vi "Count_if_Subtrack_Is_Enough_for_Cost_F()-3.vi"(3 "[IN] Indexes for Jumps\nfrom Previous Origin":i32[](array[numeric]), 4 "[IN] Index of Problem \nPoint Inside Track":i32, 5 "[IN] Minimal Subtrack Length \n(Points without problems) for\nMaking Desicion":i32, 6 "[IN] Dot Statuses in Track":i16[](array[numeric])) -> (1 "[OUT] Index of Last \nPoint in Track":i32, 2 "[OUT] It's enough to make\nconclusion using subtrack":bool)   [LabVIEW 2013]
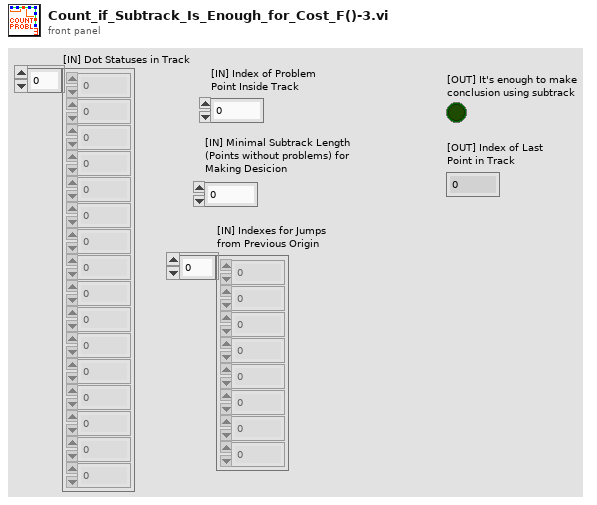
[diagram p1: front panel]
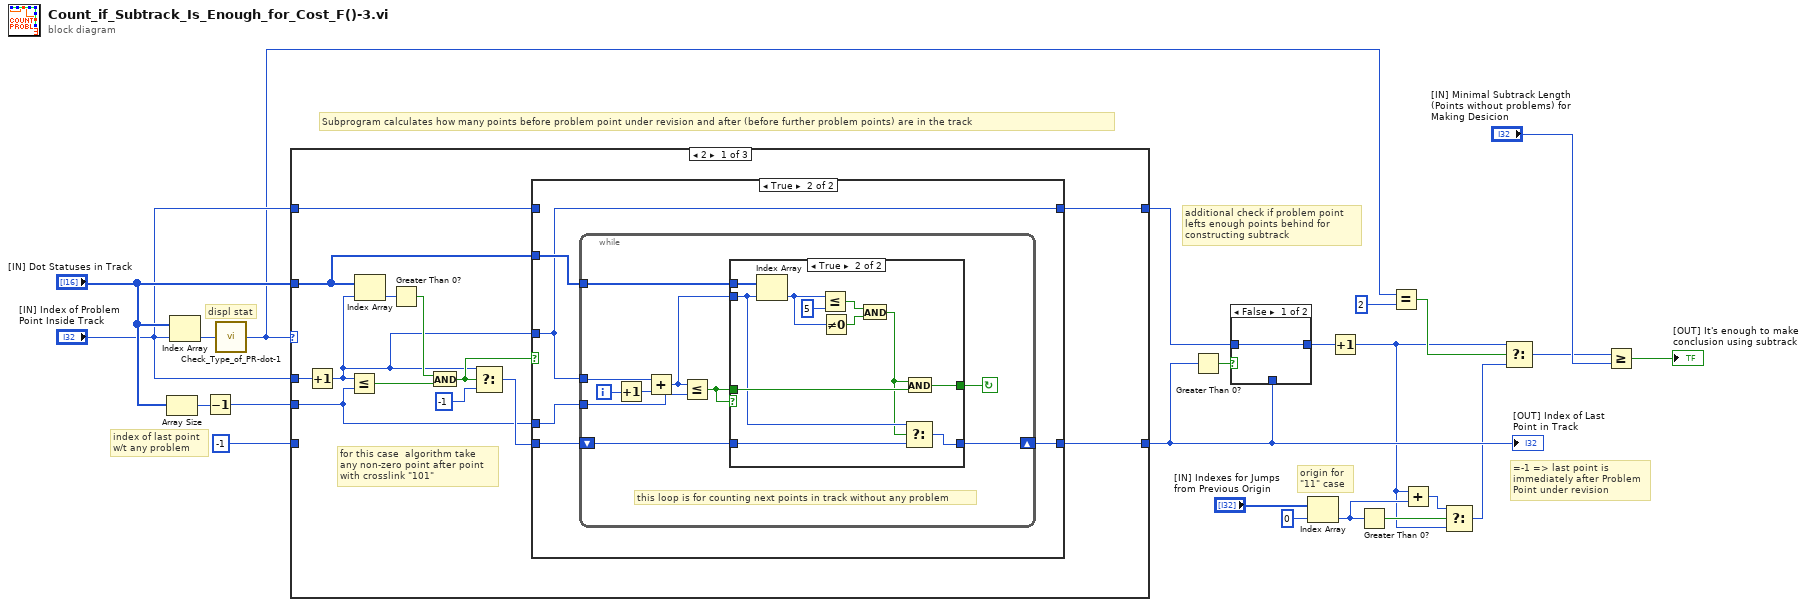
[diagram p0: block diagram]
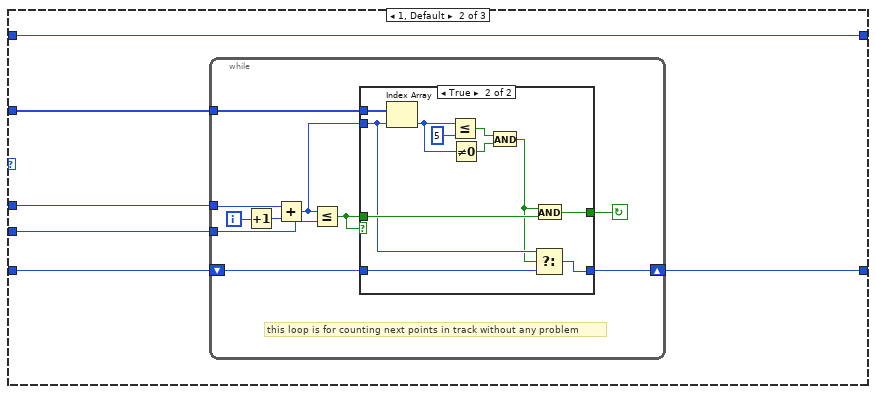
[diagram p4: hidden frame]
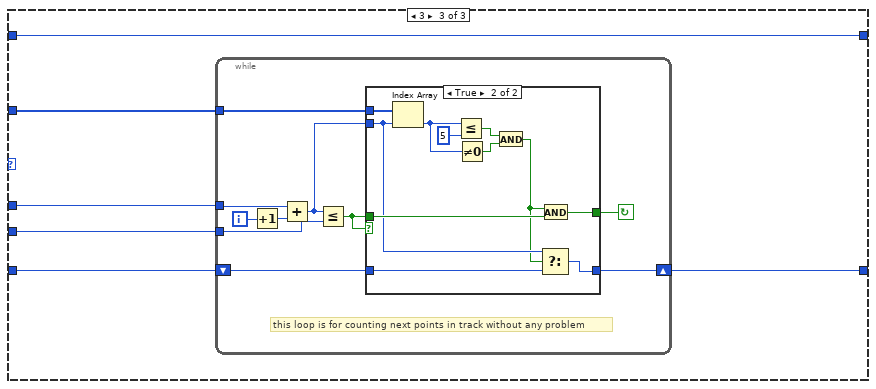
[diagram p6: hidden frame]
diagram:
  # "origin for \n\"11\" case"
  # "displ stat"
  # "additional check if problem point \nlefts enough points behind for \nconstructing subtrack"
  # "=-1 => last point is\nimmediately after Problem \nPoint under revision"
  # "Subprogram calculates how many points before problem point under revision and after (before further problem points) are in the track"
  # "index of last point\nw/t any problem"
  n1 = Array Size(array="[IN] Dot Statuses in Track") -> (size(s)=w23:i32)
  n2 = Index Array(array="[IN] Dot Statuses in Track", index="[IN] Index of Problem \nPoint Inside Track") -> (element=w15:i16)
  n3 = Decrement(x=w23) -> (x-1=w22:i32)
  n4 = call "Check_Type_of_PR-dot-1.vi"("[IN] dot status"=w15) -> ("[OUT] Type of\nproblem dot"=w10:i32)
  n5 = case shown="2" w10 {
    tunnel: w22 -> [w26 w72 w99]
    tunnel: -1 -> [_ w71 w98]
    tunnel: [w27 w70 w97] -> w17
    tunnel: "[IN] Dot Statuses in Track" -> [w28 w69 w101]
    tunnel: "[IN] Index of Problem \nPoint Inside Track" -> [w36 w68 w100]
    tunnel: "[IN] Index of Problem \nPoint Inside Track" -> [w24 w67 w96]
    tunnel: [w25 w67 w96] -> w13
    frame 2 {
      # "for this case  algorithm take\nany non-zero point after point\nwith crosslink \"101\""
      n6 = Increment(x=w36) -> (x+1=w29:i32)
      n7 = Less Or Equal?(x=w29, y=w26) -> (x <= y?=w34:bool)
      n8 = Index Array(array=w28, index=w29) -> (element=w35:i16)
      n9 = Greater Than 0?(x=w35) -> (x > 0?=w33:bool)
      n10 = And(x=w33, y=w34) -> (x .and. y?=w31:bool)
      n11 = Select(t=w29, s=w31, f=-1) -> (s? t:f=w30:i32)
      n12 = case shown="True" w31 {
        tunnel: w30 -> [w38 w43]
        tunnel: w29 -> [_ w39]
        tunnel: w28 -> [_ w42]
        tunnel: [w38 w41] -> w27
        tunnel: w26 -> [_ w40]
        tunnel: [w37 w39] -> w25
        tunnel: w24 -> [w37 _]
        frame False {
        }
        frame True {
          n13 = while {
            tunnel: w40 -> [w51]
            tunnel: w39 -> [w44]
            tunnel: w42 -> [w50]
            shift-right: [w45] -> w41
            shift-left: w43 -> [w46]
            i -> [w53]
            stop <- w47 continue-if-true
            # "this loop is for counting next points in track without any problem"
            n14 = Increment(x=w53) -> (x+1=w52:i32)
            n15 = Add(x=w44, y=w52) -> (x+y=w49:i32)
            n16 = Less Or Equal?(x=w49, y=w51) -> (x <= y?=w48:bool)
            n17 = case shown="True" w48 {
              tunnel: w50 -> [_ w66]
              tunnel: w49 -> [_ w57]
              tunnel: w48 -> [w55 w60]
              tunnel: [w55 w61] -> w47
              tunnel: w46 -> [w54 w58]
              tunnel: [w54 w59] -> w45
              frame False {
                # "it's last point in subtrack"
              }
              frame True {
                n18 = Index Array(array=w66, index=w57) -> (element=w64:i16)
                n19 = Less Or Equal?(x=w64, y=i16 5) -> (x <= y?=w63:bool)
                n20 = Not Equal To 0?(x=w64) -> (x != 0?=w62:bool)
                n21 = And(x=w63, y=w62) -> (x .and. y?=w56:bool)
                n22 = Select(t=w57, s=w56, f=w58) -> (s? t:f=w59:i32)
                n23 = And(x=w56, y=w60) -> (x .and. y?=w61:bool)
              }
            }
          }
        }
      }
    }
    frame 1, Default {
      n24 = while {
        tunnel: w72 -> [w80]
        tunnel: w68 -> [w73]
        tunnel: w69 -> [w79]
        shift-right: [w74] -> w70
        shift-left: w71 -> [w75]
        i -> [w82]
        stop <- w76 continue-if-true
        # "this loop is for counting next points in track without any problem"
        n25 = Increment(x=w82) -> (x+1=w81:i32)
        n26 = Add(x=w73, y=w81) -> (x+y=w78:i32)
        n27 = Less Or Equal?(x=w78, y=w80) -> (x <= y?=w77:bool)
        n28 = case shown="True" w77 {
          tunnel: w79 -> [_ w95]
          tunnel: w78 -> [_ w86]
          tunnel: w77 -> [w84 w89]
          tunnel: [w84 w90] -> w76
          tunnel: w75 -> [w83 w87]
          tunnel: [w83 w88] -> w74
          frame False {
            # "it's last point in subtrack"
          }
          frame True {
            n29 = Index Array(array=w95, index=w86) -> (element=w93:i16)
            n30 = Less Or Equal?(x=w93, y=i16 5) -> (x <= y?=w92:bool)
            n31 = Not Equal To 0?(x=w93) -> (x != 0?=w91:bool)
            n32 = And(x=w92, y=w91) -> (x .and. y?=w85:bool)
            n33 = Select(t=w86, s=w85, f=w87) -> (s? t:f=w88:i32)
            n34 = And(x=w85, y=w89) -> (x .and. y?=w90:bool)
          }
        }
      }
    }
    frame 3 {
      n35 = while {
        tunnel: w99 -> [w109]
        tunnel: w100 -> [w102]
        tunnel: w101 -> [w108]
        shift-right: [w103] -> w97
        shift-left: w98 -> [w104]
        i -> [w111]
        stop <- w105 continue-if-true
        # "this loop is for counting next points in track without any problem"
        n36 = Increment(x=w111) -> (x+1=w110:i32)
        n37 = Add(x=w102, y=w110) -> (x+y=w107:i32)
        n38 = Less Or Equal?(x=w107, y=w109) -> (x <= y?=w106:bool)
        n39 = case shown="True" w106 {
          tunnel: w108 -> [_ w124]
          tunnel: w107 -> [_ w115]
          tunnel: w106 -> [w113 w118]
          tunnel: [w113 w119] -> w105
          tunnel: w104 -> [w112 w116]
          tunnel: [w112 w117] -> w103
          frame False {
            # "it's last point in subtrack"
          }
          frame True {
            n40 = Index Array(array=w124, index=w115) -> (element=w122:i16)
            n41 = Less Or Equal?(x=w122, y=i16 5) -> (x <= y?=w121:bool)
            n42 = Not Equal To 0?(x=w122) -> (x != 0?=w120:bool)
            n43 = And(x=w121, y=w120) -> (x .and. y?=w114:bool)
            n44 = Select(t=w115, s=w114, f=w116) -> (s? t:f=w117:i32)
            n45 = And(x=w114, y=w118) -> (x .and. y?=w119:bool)
          }
        }
      }
    }
  }
  "[OUT] Index of Last \nPoint in Track" <- w17
  n46 = Greater Than 0?(x=w17) -> (x > 0?=w19:bool)
  n47 = case shown="False" w19 {
    tunnel: w13 -> [w125 _]
    tunnel: [w125 w126] -> w18
    tunnel: w17 -> [_ w126]
    frame False {
    }
    frame True {
    }
  }
  n48 = Index Array(array="[IN] Indexes for Jumps\nfrom Previous Origin", index=0) -> (element=w4:i32)
  n49 = Increment(x=w18) -> (x+1=w2:i32)
  n50 = Greater Than 0?(x=w4) -> (x > 0?=w5:bool)
  n51 = Equal?(x=w10, y=2) -> (x = y?=w8:bool)
  n52 = Add(x=w2, y=w4) -> (x+y=w3:i32)
  n53 = Select(t=w3, s=w5, f=w2) -> (s? t:f=w1:i32)
  n54 = Select(t=w2, s=w8, f=w1) -> (s? t:f=w7:i32)
  n55 = Greater Or Equal?(x=w7, y="[IN] Minimal Subtrack Length \n(Points without problems) for\nMaking Desicion") -> (x >= y?=→"[OUT] It's enough to make\nconclusion using subtrack":bool)
